vi "OpenReferencedVI.vi"(9 "CThread Reference":refnum<vi>, 19 "error in (no error)":errorcluster) -> (8 "VI Name":string, 10 "VI Path":path, 12 "Clone":i16, 14 "Encoded Name":u32, 18 "error out":errorcluster)   [LabVIEW 2012, in "CThread.lvlib"]
uses:
  CThread.lvlib
panel:
  out "Clone Number (-1)":i16
  out "vi reference":refnum<vi>
  in  "VI Reference":string
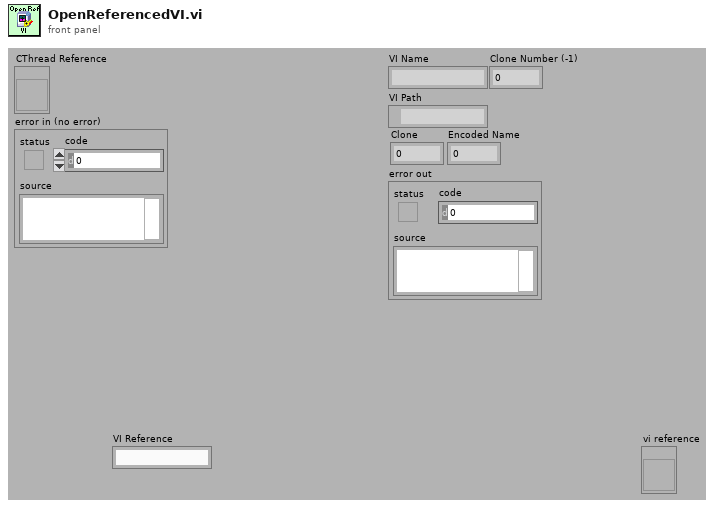
[diagram p1: front panel]
types:
  T1 = typedef "CThread.lvlib/CThread VI Reference.xnode/State.ctl" = cluster{"VI Name":string, "VI Path":path, "Clone":i16, "Encoded Name":u32}
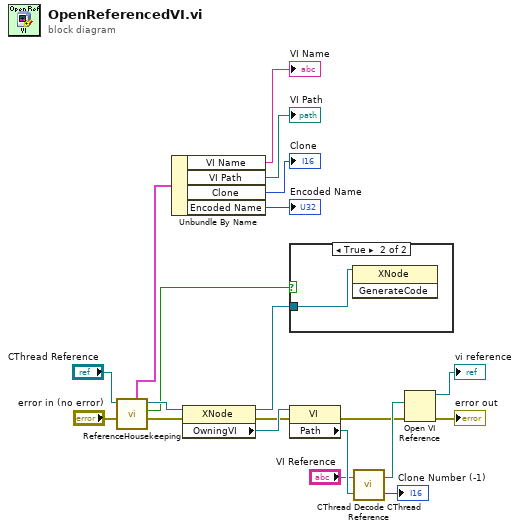
[diagram p0: block diagram]
diagram:
  n1 = call "ReferenceHousekeeping.vi"("error in (no error)"="error in (no error)", "CThread Reference"="CThread Reference") -> ("error out"=w1:errorcluster, "Modified?"=w5:bool, "XRef Out"=w9:refnum<vi>, "State Out"=w8:T1)  [unwired: 6 in]
  n2 = Unbundle By Name(w8) -> ("VI Name"=→"VI Name":string, "VI Path"=→"VI Path":path, "Clone"=→"Clone":i16, "Encoded Name"=→"Encoded Name":u32)
  n3 = property class="XNode"(reference=w9, error in=w1) -> (reference out=w3:refnum<vi>, error out=w15:errorcluster, "OwningVI"=w16:refnum<vi>)
  n4 = case shown="True" w5 {
    tunnel: w3 -> [_ w21]
    frame False {
    }
    frame True {
      n5 = invoke class="XNode" method="GenerateCode"(reference=w21) -> ()  [unwired: 2 in, 3 out]
    }
  }
  n6 = property class="VI"(reference=w16, error in=w15) -> (error out=w12:errorcluster, "Path"=w14:path)  [unwired: 1 out]
  n7 = call "CThread Decode CThread Reference.vi"("Owner Path"=w14, "CThread Reference"="VI Reference") -> ("Clone Number"=→"Clone Number (-1)":i16, "path"=w13:path)
  n8 = Open VI Reference(vi path=w13, error in (no error)=w12) -> (vi reference=→"vi reference":refnum<vi>, error out=→"error out":errorcluster)  [unwired: 4 in]
